vi "Send-command.vi"(8 "error in (no error)":errorcluster, 10 "Command string":string, 11 "SM1000-control in":refnum<class "SM1000-control.lvclass">) -> (0 "error out":errorcluster, 3 "SM1000-control out":refnum<class "SM1000-control.lvclass">)   [LabVIEW 2013, in "EC1000-control.lvlib" / "SM1000-control.lvclass"]
uses:
  SM1000-control.lvclass
  SM1000-control.lvclass/SM1000-control.ctl
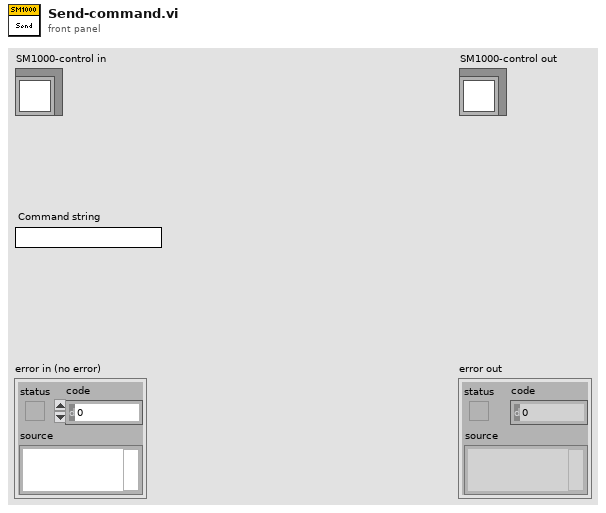
[diagram p1: front panel]
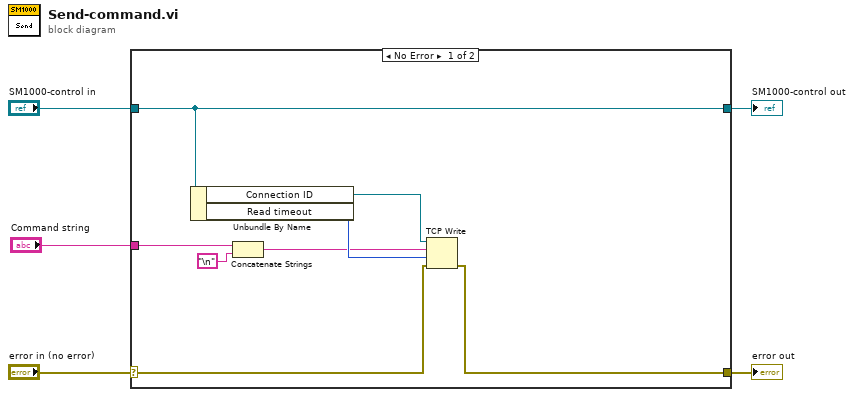
[diagram p0: block diagram]
diagram:
  n1 = case shown="No Error" "error in (no error)" {
    selector: "error in (no error)" -> [w9 w15]
    tunnel: [w8 w15] -> w4
    tunnel: [w13 w14] -> w2
    tunnel: "SM1000-control in" -> [w13 w14]
    tunnel: "Command string" -> [w11 _]
    frame No Error {
      n2 = Unbundle By Name(w13) -> ("Connection ID"=w12:refnum<k5>, "Read timeout"=w10:i32)
      n3 = Concatenate Strings(w11, "\n") -> (w7:string)
      n4 = TCP Write(connection ID=w12, data in=w7, error in (no error)=w9, 9:w10) -> (error out=w8:errorcluster)  [unwired: 2 out]
    }
    frame Error {
    }
  }
  "error out" <- w4
  "SM1000-control out" <- w2
